vi "Close.vi"(8 "error in (no error)":errorcluster, 11 "Communication in":refnum<class "Network.lvclass">) -> (0 "error out":errorcluster, 3 "Communication out":refnum<class "Network.lvclass">)   [LabVIEW 2020, in "Communication Classes.lvlib" / "Network.lvclass"]
uses:
  Network.lvclass
  IP_Communication/IP_Communication.lvclass
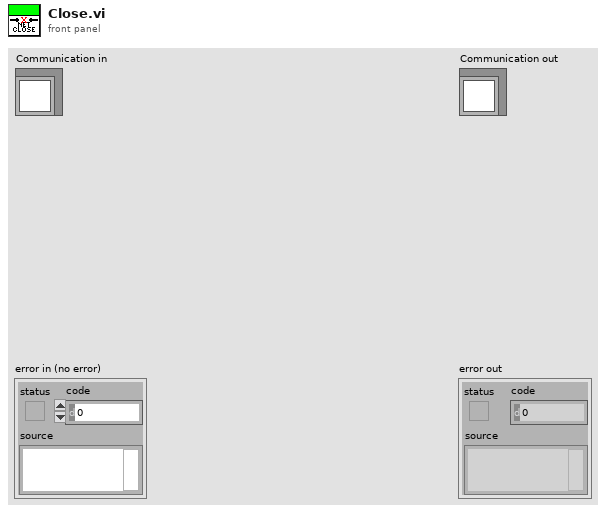
[diagram p1: front panel]
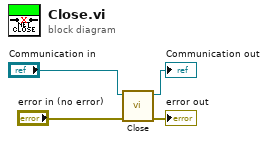
[diagram p0: block diagram]
diagram:
  n1 = call-parent "Close.vi"("error in (no error)"="error in (no error)", "Communication in"="Communication in") -> ("error out"=→"error out":errorcluster, "Communication out"=→"Communication out":refnum<class "Network.lvclass">)  [unwired: 8 in]
